vi "Write Delay.vi"(8 "error in (no error)":errorcluster, 10 "Delay":i32, 11 "Macro Step in":refnum<class "Macro Step.lvclass">) -> (0 "error out":errorcluster, 3 "Macro Step out":refnum<class "Macro Step.lvclass">)   [LabVIEW 2020, in "MacroAssert.lvlib" / "Macro Step.lvclass"]
uses:
  Macro Step.lvclass
  Macro Step.lvclass/Macro Step.ctl
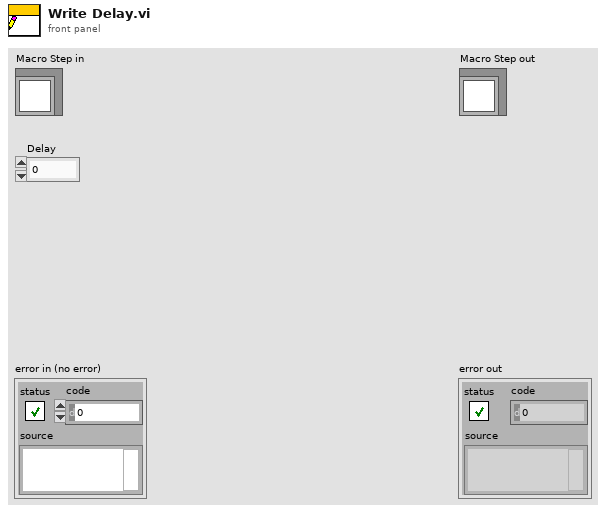
[diagram p1: front panel]
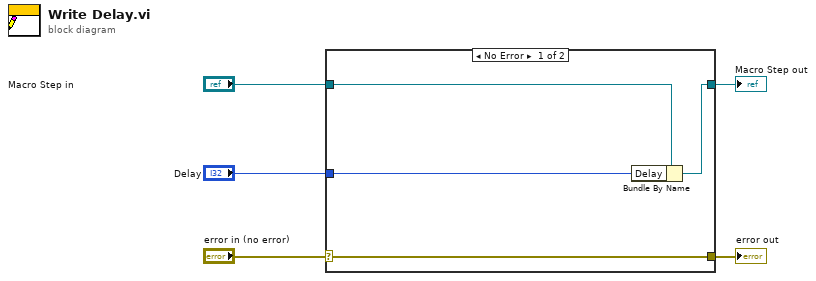
[diagram p0: block diagram]
diagram:
  n1 = case shown="No Error" "error in (no error)" {
    selector: "error in (no error)" -> [w9 w10]
    tunnel: [w9 w10] -> w4
    tunnel: [w7 w11] -> w2
    tunnel: "Macro Step in" -> [w8 w11]
    tunnel: "Delay" -> [w6 _]
    frame No Error {
      n2 = Bundle By Name(cluster=w8, "Delay"=w6) -> (w7:refnum<class "Macro Step.lvclass">)
    }
    frame Error {
    }
  }
  "error out" <- w4
  "Macro Step out" <- w2
